vi "CalcXValue(SubVI).vi"(11 "CrsrList":T1) -> (1 "Line 2 A":dbl, 3 "Line 1 A":dbl, 5 "X-value":dbl)   [LabVIEW 2013, in "main.lvlib"]
uses:
  main.lvlib
  <vilib>/Utility/miscctls.llb/LVCursorListTypeDef.ctl
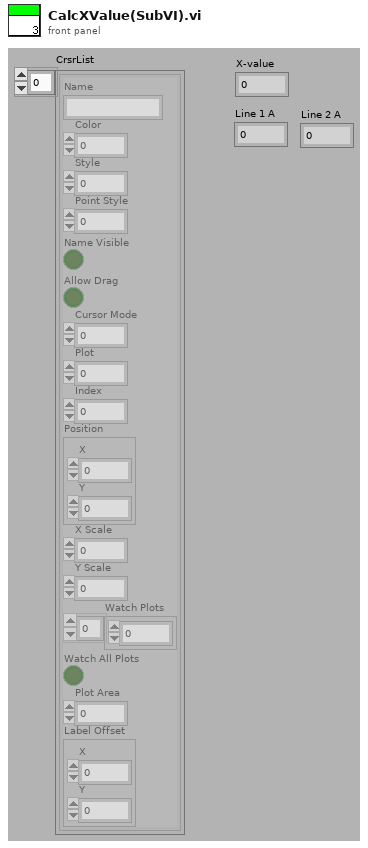
[diagram p1: front panel]
types:
  T1 = typedef "LVCursorListTypeDef.ctl" = cluster{"Name":string, "Color":u32, "Style":u8, "Point Style":u8, "Name Visible":bool, "Allow Drag":bool, "Cursor Mode":u32, "Plot":i32, "Index":i32, "Position":cluster{"X":dbl, "Y":dbl}, "X Scale":u32, "Y Scale":u32, "Watch Plots":i32[], "Watch All Plots":bool, "Plot Area":i32, "Label Offset":cluster{"X":dbl, "Y":dbl}}[]
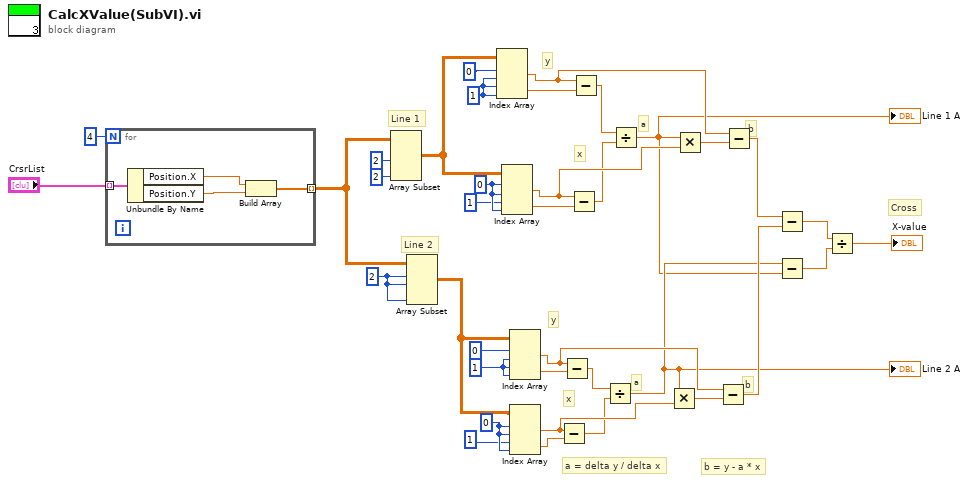
[diagram p0: block diagram]
diagram:
  w16 = 0
  w15 = 0
  w10 = 1 ("index (row)")
  w8 = 1 ("index (row)")
  w7 = 2
  # "b = y - a * x"
  # "a = delta y / delta x"
  # "Cross"
  # "b"
  # "a"
  # "b"
  # "a"
  # "Line 2"
  # "Line 1"
  # "y"
  # "x"
  # "x"
  # "y"
  n1 = for {
    N: 4 -> [_]
    tunnel: "CrsrList" -> [w41] mode=indexing
    tunnel: [w39] -> w19 mode=indexing
    n2 = Unbundle By Name(w41) -> ("Position.X"=w38:dbl, "Position.Y"=w40:dbl)
    n3 = Build Array(w38, w40) -> (w39:dbl[])
  }
  n4 = Array Subset(array=w19, length (row)=2 ("length"), length (col)=2 ("length")) -> (w17:dbl[][])  [unwired: 2 in]
  n5 = Array Subset(array=w19, index (row)=w7, length (row)=w7, length (col)=w7) -> (w18:dbl[][])  [unwired: 1 in]
  n6 = Index Array(array=w17, index (row) #1=0 ("disabled index (col)"), index (col) #1=w8, index (row) #2=w8, index (col) #2=w8) -> (element #1=w23:dbl, element #2=w24:dbl)
  n7 = Index Array(array=w17, index (row) #1=w16, index (col) #1=w16, index (row) #2=1 ("index"), index (col) #2=w16) -> (element #1=w26:dbl, element #2=w25:dbl)
  n8 = Index Array(array=w18, index (row) #1=0 ("index (row)"), index (col) #1=w10, index (row) #2=w10, index (col) #2=w10) -> (element #1=w37:dbl, element #2=w6:dbl)
  n9 = Index Array(array=w18, index (row) #1=w15, index (col) #1=w15, index (row) #2=1 ("index"), index (col) #2=w15) -> (element #1=w30:dbl, element #2=w12:dbl)
  n10 = Subtract(x=w30, y=w12) -> (x-y=w28:dbl)
  n11 = Subtract(x=w37, y=w6) -> (x-y=w29:dbl)
  n12 = Subtract(x=w26, y=w25) -> (x-y=w21:dbl)
  n13 = Subtract(x=w23, y=w24) -> (x-y=w20:dbl)
  n14 = Divide(x=w29, y=w28) -> (x/y=w34:dbl)
  "Line 2 A" <- w34
  n15 = Divide(x=w20, y=w21) -> (x/y=w1:dbl)
  "Line 1 A" <- w1
  n16 = Multiply(x=w34, y=w30) -> (x*y=w27:dbl)
  n17 = Multiply(x=w1, y=w26) -> (x*y=w22:dbl)
  n18 = Subtract(x=w37, y=w27) -> (x-y=w36:dbl)
  n19 = Subtract(x=w23, y=w22) -> (x-y=w35:dbl)
  n20 = Subtract(x=w35, y=w36) -> (x-y=w31:dbl)
  n21 = Subtract(x=w34, y=w1) -> (x-y=w32:dbl)
  n22 = Divide(x=w31, y=w32) -> (x/y=→"X-value":dbl)
